vi "Wait.vi"(4 "error in (no error)":errorcluster caption="错误输入（无错误）", 7 "Delay(100ms)":u32=100) -> (0 "error out":errorcluster caption="错误输出")   [LabVIEW 2020]
doc: "该模板用于创建子VI。"
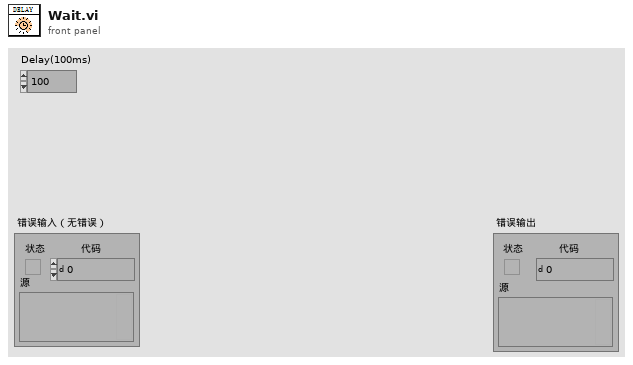
[diagram p1: front panel]
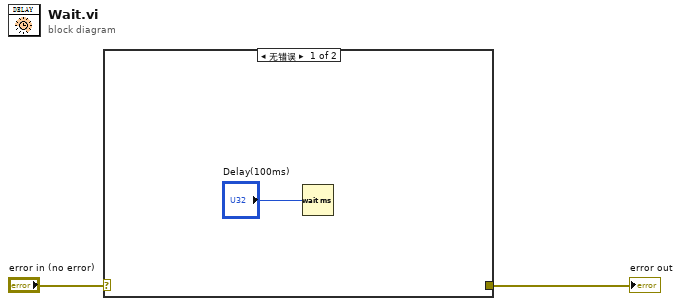
[diagram p0: block diagram]
diagram:
  n1 = case shown="无错误" "error in (no error)" {
    selector: "error in (no error)" -> [_ w4]
    tunnel: [_ w4] -> w1
    frame No Error {
      n2 = Wait (ms)(milliseconds to wait="Delay(100ms)") -> ()  [unwired: 1 out]
    }
    frame Error {
    }
  }
  "error out" <- w1
